vi "GetType.vi"(8 "error in (no error)":errorcluster, 11 "Configure Advanced Trigger [AT] Msg in":refnum<class "Configure Advanced Trigger [AT] Msg.lvclass">) -> (0 "error out":errorcluster, 2 "Data Sample":variant, 3 "Configure Advanced Trigger [AT] Msg out":refnum<class "Configure Advanced Trigger [AT] Msg.lvclass">)   [LabVIEW 2014, in "CS++Fgen.lvlib" / "Configure Advanced Trigger [AT] Msg.lvclass"]
doc: "This VI delivers a sample of the data type format the message expects."
uses:
  Configure Advanced Trigger [AT] Msg.lvclass
  Configure Advanced Trigger [AT] Msg.lvclass/Configure Advanced Trigger [AT] Msg.ctl
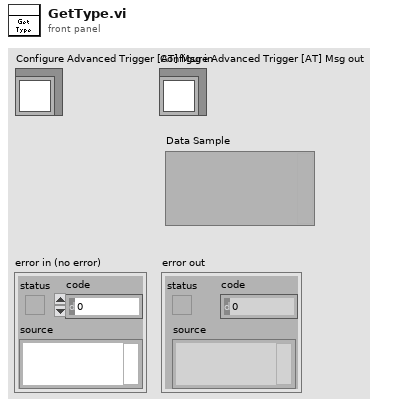
[diagram p1: front panel]
types:
  T1 = cluster{"Trigger Slope (Positive)":i32, "Channel Name (\"\")":string, "Trigger Source (None)":string}
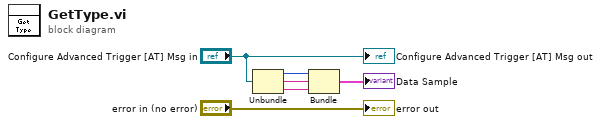
[diagram p0: block diagram]
diagram:
  n1 = Unbundle("Configure Advanced Trigger [AT] Msg in") -> (w4:i32, w3:string, w2:string)
  n2 = Bundle("Trigger Slope (Positive)"=w4, "Channel Name (\"\")"=w3, "Trigger Source (None)"=w2) -> (→"Data Sample":T1)  [unwired: 1 in]
  "error out" <- "error in (no error)"
  "Configure Advanced Trigger [AT] Msg out" <- "Configure Advanced Trigger [AT] Msg in"
